vi "Self Configure.vi"(8 "error in":errorcluster, 11 "4300 in":refnum<class "4300.lvclass">) -> (0 "error out":errorcluster, 3 "4300 out":refnum<class "4300.lvclass">)   [LabVIEW 2019, in "4300.lvlib" / "4300.lvclass"]
uses:
  Library/4300.lvclass
  C:/Users/Public/Documents/Development/builds/Instruments/Instruments.lvlibp/Library/Instruments.lvclass
  builds/Instruments/Instruments.lvlibp/Accessors/Write Padding_enable.vi
  builds/Instruments/AnalogInput.lvlibp/Library/AnalogInput.lvclass
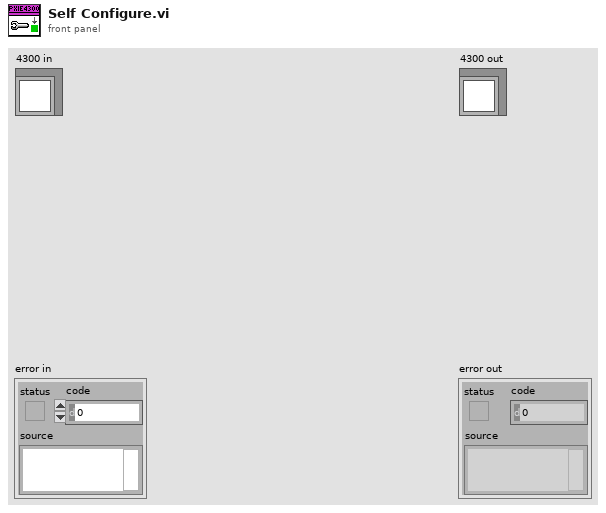
[diagram p1: front panel]
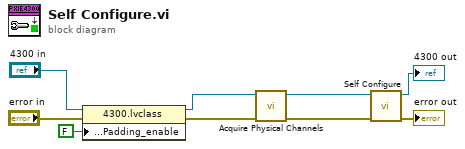
[diagram p0: block diagram]
diagram:
  n1 = property class="4300.lvclass"(reference="4300 in", error in="error in", "Accessors:Logging:Padding_enable"=FALSE ("Instrument:Logging:Padding:Enable")) -> (reference out=w4:refnum<class "4300.lvclass">, error out=w3:errorcluster)
  n2 = call "Acquire Physical Channels.vi"("error in"=w3, "4300 in"=w4) -> ("error out"=w2:errorcluster, "4300 out"=w1:refnum<class "4300.lvclass">)  [unwired: 8 in]
  n3 = call-parent "Self Configure.vi"("error in"=w2, "AnalogInput in"=w1) -> ("error out"=→"error out":errorcluster, "AnalogInput out"=→"4300 out":refnum<class "4300.lvclass">)  [unwired: 8 in]
